vi "Video_1.vi"() -> ()   [LabVIEW 2012]
uses:
  SubVIs/LVPresent_Globals.vi
  <vilib>/Platform/browser.llb/Open URL in Default Browser (string).vi
panel:
  in  "Play Video here!":bool
  # "Intro to LabVIEW Video\n\nClick the button below to open a link to the JumboBooks website. Please watch the Intro to LabVIEW Video before proceeding onto the next slide."
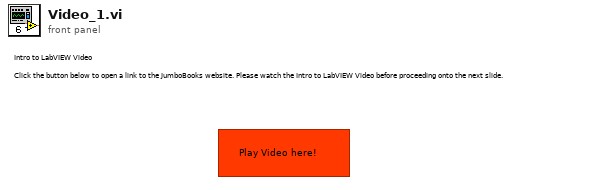
[diagram p1: front panel]
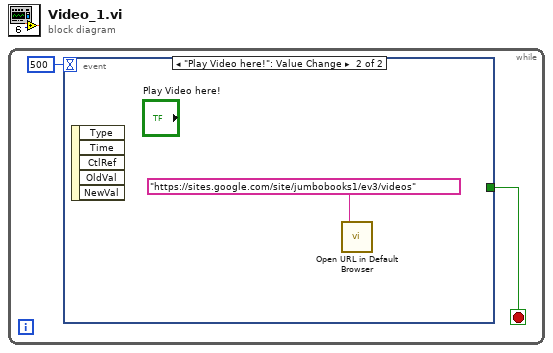
[diagram p0: block diagram]
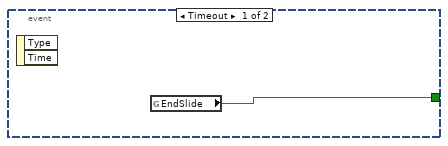
[diagram p2: hidden frame]
diagram:
  n1 = while {
    stop <- w2 stop-if-true
    n2 = event shown="[1] \"Play Video here!\": Value Change" {
      selector: _ -> [_ _]
      dyn-events: _ -> [_ _]
      timeout: 500 -> [_ _]
      tunnel: [w3 _] -> w2
      event Timeout {
        n3 = event-data() -> ()  [unwired: 1 in, 2 out]
        n4 = global read "LVPresent_Globals.vi" "EndSlide"() -> (w3:bool)
      }
      event "Play Video here!": Value Change {
        n5 = event-data() -> ()  [unwired: 1 in, 5 out]
        n6 = call-poly <vilib>:"Open URL in Default Browser.vi"("URL"="https://sites.google.com/site/jumbobooks1/ev3/videos") -> ()  [unwired: 5 in, 2 out]
      }
    }
  }
